vi "List Auto Col Length.vi"   [LabVIEW 2014]
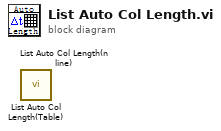
[diagram p0: block diagram]
diagram:
  n1 = call "List Auto Col Length(Table).vi"() -> ()  [unwired: 10 in, 2 out]
  n2 = call "List Auto Col Length(n line).vi"() -> ()  [unwired: 10 in, 2 out]
